vi "PV DHW Temperature Conversion.vi"(11 "HEX Data Array (Temp)":u8[](array[numeric]) format="%.0x") -> (3 "DHW Temp (°F)":string)   [LabVIEW 2023]
panel:
  out "(hi.lo)":u16 format="%x"
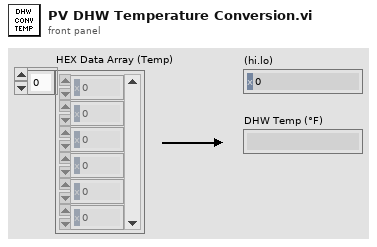
[diagram p1: front panel]
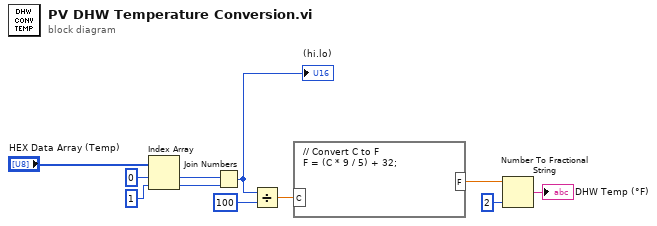
[diagram p0: block diagram]
diagram:
  n1 = Index Array(array="HEX Data Array (Temp)", index #1=0 ("index"), index #2=1 ("index")) -> (element #1=w2:u8, element #2=w1:u8)
  n2 = Join Numbers(hi=w2, lo=w1) -> ((hi.lo)=w9:u16)
  "(hi.lo)" <- w9
  n3 = Divide(x=w9, y=u16 100) -> (x/y=w11:dbl)
  n4 = formula code="// Convert C to F\nF = (C * 9 / 5) + 32;"("C"=w11) -> ("F"=w8:dbl)
  n5 = Number To Fractional String(number=w8, precision (6)=i16 2) -> (F-format string=→"DHW Temp (°F)":string)  [unwired: 2 in]
